vi "Workorder DB Operation.vi"(6 "create batch":T1, 7 "WO OP":T3, 8 "error in (no error)":errorcluster, 9 "Status":T2, 10 "Workorder name":string, 11 "REF in":T4) -> (0 "error out":errorcluster, 1 "Success":bool, 2 "Open batch":T1, 3 "REF out":T4, 4 "paused and ready WOs":string[](array[string]))   [LabVIEW 2024]
uses:
  CTRLS/REF.ctl
  CTRLS/Main Tabs.ctl
  CTRLS/Open Batch Data.ctl
  CTRLS/DM_Data.ctl
  CTRLS/run statistics.ctl
  CTRLS/System settings.ctl
  CTRLS/Printer Message settings.ctl
  CTRLS/Workorder DB operation enum.ctl
  CTRLS/Workorder status enum.ctl
  CTRLS/DB operation Selector.ctl
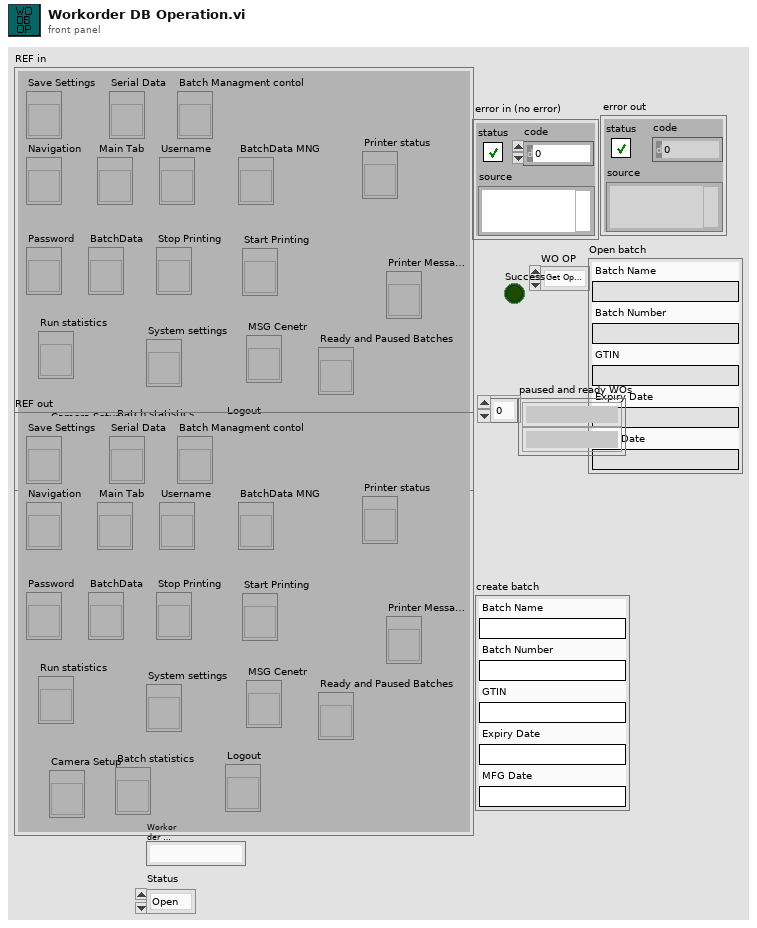
[diagram p1: front panel]
types:
  T1 = typedef "Open Batch Data.ctl" = cluster{"Batch Name":string, "Batch Number":string, "GTIN":string, "Expiry Date":string, "MFG Date":string}
  T2 = typedef "Workorder status enum.ctl" = enum16{"Open", "Ready", "On Hold", "Closed"}
  T3 = typedef "Workorder DB operation enum.ctl" = enum16{"Get Open Workorder", "Change WO Status", "Create WO", "Get ready and paused WOs"}
  T4 = typedef "REF.ctl" = cluster{"Save Settings":refnum<vi>, "Navigation":refnum<vi>, "Main Tab":refnum<vi>, "Password":refnum<vi>, "BatchData":refnum<vi>, "Serial Data":refnum<vi>, "Username":refnum<vi>, "Stop Printing":refnum<vi>, "Run statistics":refnum<vi>, "System settings":refnum<vi>, "Batch Managment contol":refnum<vi>, "Start Printing":refnum<vi>, "BatchData MNG":refnum<vi>, "MSG Cenetr":refnum<vi>, "Printer status":refnum<vi>, "Printer Message Config":refnum<vi>, "Ready and Paused Batches":refnum<vi>, "Camera Setup":refnum<vi>, "Batch statistics":refnum<vi>, "Logout":refnum<vi>}
  T5 = typedef "NI_Database_API.lvlib/Conn ObjectReference.ctl" = refnum<k1>
  T6 = typedef "DB operation Selector.ctl" = enum16{"Select", "Insert", "Update", "Execute select Query", "Execute update query"}
  T7 = cluster{"Batch Name":string, "Batch Number":string, "GTIN":string, "Expiry Date":string, "MFG Date":string, string}
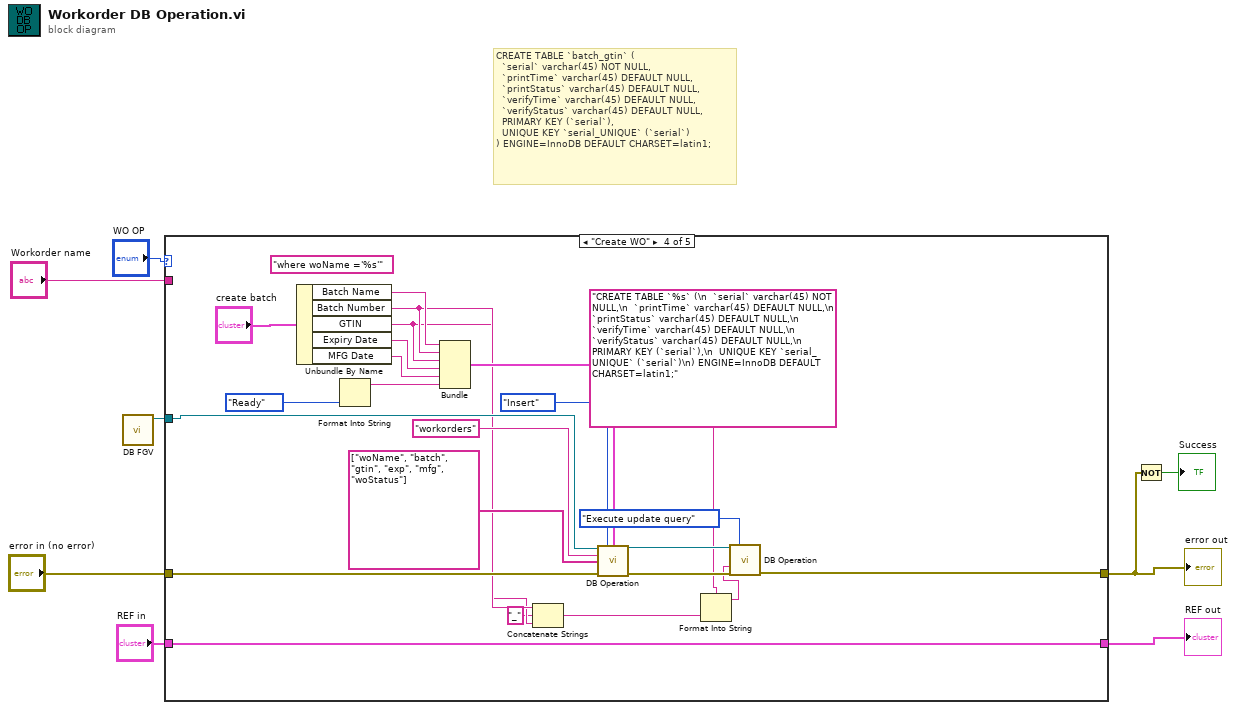
[diagram p0: block diagram]
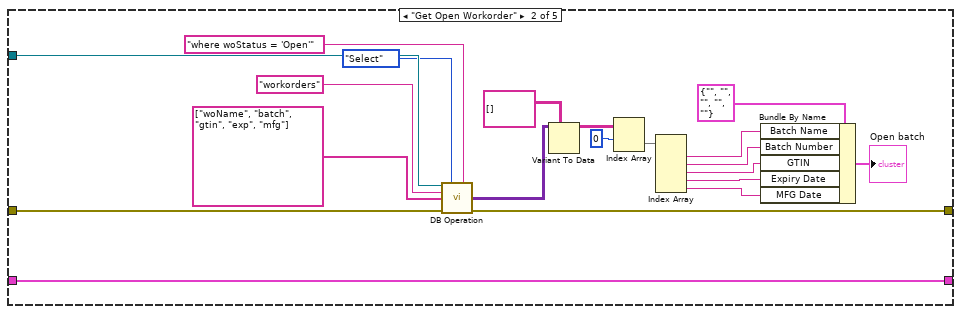
[diagram p3: hidden frame]
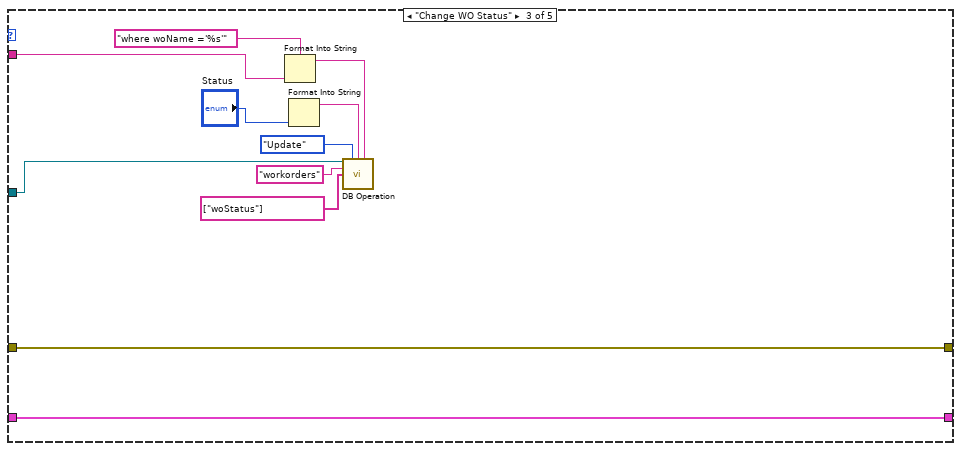
[diagram p4: hidden frame]
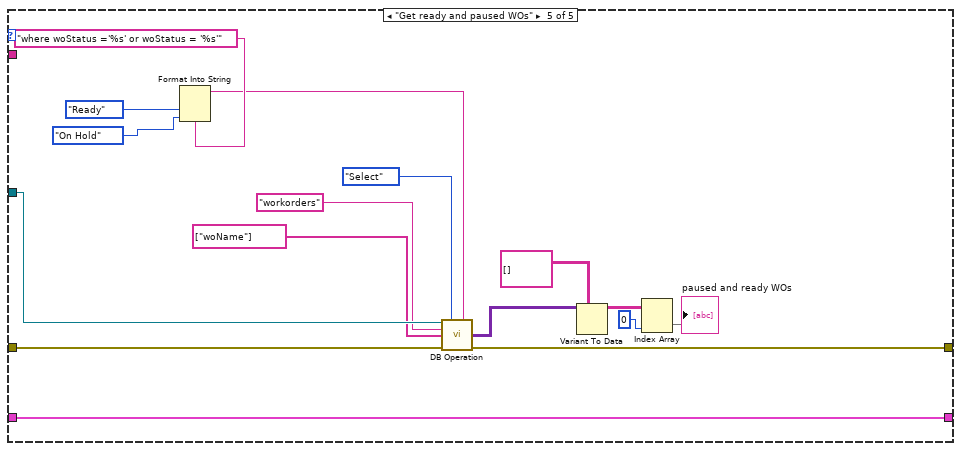
[diagram p5: hidden frame]
diagram:
  # "CREATE TABLE `batch_gtin` (\n  `serial` varchar(45) NOT NULL,\n  `printTime` varchar(45) DEFAULT NULL,\n  `printStatus` varchar(45) DEFAULT NULL,\n  `verifyTime` varchar(45) DEFAULT NULL,\n  `verifyStatus` varchar(45) DEFAULT NULL,\n  PRIMARY KEY (`serial`),\n  UNIQUE KEY `serial_UNIQUE` (`serial`)\n) ENGINE=InnoDB DEFAULT CHARSET=latin1;"
  n1 = call "DB FGV.vi"() -> ("DB ref"=w7:T5)  [unwired: 11 in]
  n2 = case shown="\"Create WO\"" "WO OP" {
    tunnel: w7 -> [_ w30 w39 w63 w79]
    tunnel: "error in (no error)" -> [w10 w27 w41 w59 w75]
    tunnel: [w10 w26 w41 w42 w74] -> w2
    tunnel: [w9 w19 w40 w64 w80] -> w5
    tunnel: "REF in" -> [w9 w19 w40 w64 w80]
    tunnel: "Workorder name" -> [_ _ w37 _ _]
    frame Default {
    }
    frame "Get Open Workorder" {
      n3 = call "DB Operation.vi"("connection reference"=w30, "DB Op Selector"=DB_operation_Selector."Select", "Condition"="where woStatus = 'Open'", "table"="workorders", "columns"=string[] ["woName", "batch", "gtin", "exp", "mfg"], "error in (no error)"=w27) -> ("data out"=w22:variant[][], "error out"=w26:errorcluster)  [unwired: 7 in, 1 out]
      n4 = Variant To Data(type=string[][] [], Variant=w22) -> (data=w21:string[][])  [unwired: 1 in, 1 out]
      n5 = Index Array(array=w21, index (row)=0) -> (element=w16:string[])  [unwired: 1 in]
      n6 = Index Array(array=w16) -> (element #1=w15:string, element #2=w14:string, element #3=w13:string, element #4=w12:string, element #5=w11:string)  [unwired: 5 in]
      n7 = Bundle By Name(cluster=T1 {"Batch Name"="", "Batch Number"="", "GTIN"="", "Expiry Date"="", "MFG Date"=""} ("Open batch"), "Batch Name"=w15, "Batch Number"=w14, "GTIN"=w13, "Expiry Date"=w12, "MFG Date"=w11) -> (→"Open batch":T1)
    }
    frame "Change WO Status" {
      n8 = Format Into String(format string="where woName ='%s'", w37) -> (resulting string=w35:string)  [unwired: 2 in, 1 out]
      n9 = Format Into String("Status") -> (resulting string=w31:string)  [unwired: 3 in, 1 out]
      n10 = call "DB Operation.vi"("connection reference"=w39, "DB Op Selector"=DB_operation_Selector."Update", "data"=w31, "Condition"=w35, "table"="workorders", "columns"=string[] ["woStatus"]) -> ()  [unwired: 7 in, 3 out]
    }
    frame "Create WO" {
      (unwired) "where woName ='%s'" ("format string")
      n11 = Unbundle By Name("create batch") -> ("Batch Name"=w57:string, "Batch Number"=w47:string, "GTIN"=w46:string, "Expiry Date"=w56:string, "MFG Date"=w55:string)
      n12 = Format Into String(Workorder_status_enum."Ready" ("Status 2")) -> (resulting string=w53:string)  [unwired: 3 in, 1 out]
      n13 = Bundle("Batch Name"=w57, "Batch Number"=w47, "GTIN"=w46, "Expiry Date"=w56, "MFG Date"=w55, w53) -> (w52:T7)  [unwired: 1 in]
      n14 = Concatenate Strings(w47, "_" ("string"), w46) -> (w44:string)
      n15 = call "DB Operation.vi"("connection reference"=w63, "DB Op Selector"=DB_operation_Selector."Insert", "data"=w52, "table"="workorders", "columns"=string[] ["woName", "batch", "gtin", "exp", "mfg", "woStatus"], "error in (no error)"=w59) -> ("connection reference out"=w50:T5, "error out"=w51:errorcluster)  [unwired: 7 in, 1 out]
      n16 = Format Into String(format string="CREATE TABLE `%s` (\n  `serial` varchar(45) NOT NULL,\n  `printTime` varchar(45) DEFAULT NULL,\n  `printStatus` varchar(45) DEFAULT NULL,\n  `verifyTime` varchar(45) DEFAULT NULL,\n  `verifyStatus` varchar(45) DEFAULT NULL,\n  PRIMARY KEY (`serial`),\n  UNIQUE KEY `serial_UNIQUE` (`serial`)\n) ENGINE=InnoDB DEFAULT CHARSET=latin1;" ("SQL Query"), w44) -> (resulting string=w43:string)  [unwired: 2 in, 1 out]
      n17 = call "DB Operation.vi"("connection reference"=w50, "DB Op Selector"=DB_operation_Selector."Execute update query", "SQL Query"=w43, "error in (no error)"=w51) -> ("error out"=w42:errorcluster)  [unwired: 9 in, 2 out]
    }
    frame "Get ready and paused WOs" {
      n18 = Format Into String(format string="where woStatus ='%s' or woStatus = '%s'", Workorder_status_enum."Ready" ("Status 2"), Workorder_status_enum."On Hold" ("Status 2")) -> (resulting string=w70:string)  [unwired: 2 in, 1 out]
      n19 = call "DB Operation.vi"("connection reference"=w79, "DB Op Selector"=DB_operation_Selector."Select", "Condition"=w70, "table"="workorders", "columns"=string[] ["woName"], "error in (no error)"=w75) -> ("data out"=w67:variant[][], "error out"=w74:errorcluster)  [unwired: 7 in, 1 out]
      n20 = Variant To Data(type=string[][] [], Variant=w67) -> (data=w68:string[][])  [unwired: 1 in, 1 out]
      n21 = Index Array(array=w68, index (col)=0 ("index (row)")) -> (element=→"paused and ready WOs":string[])  [unwired: 1 in]
    }
  }
  "REF out" <- w5
  "error out" <- w2
  n22 = Not(x=w2) -> (.not. x?=→"Success":bool)
